vi "TableToXYGraphMot.vi"(1 "Input Table":string[][](array[string])) -> (0 "XY Graph":cluster{"Y":dbl[], "Y":dbl[]}[](graph) caption="Graphe XY")   [LabVIEW 2010]
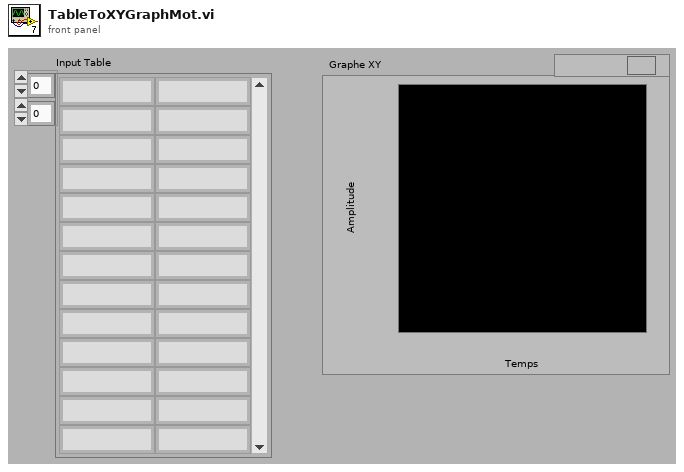
[diagram p1: front panel]
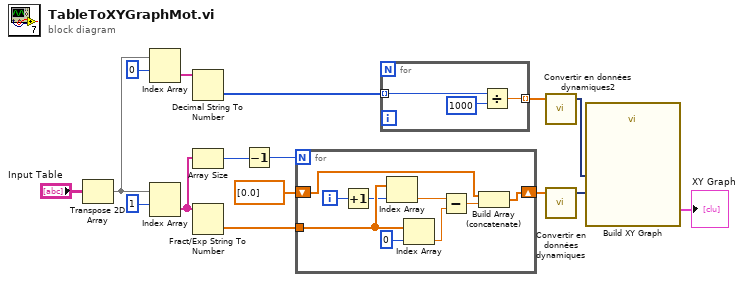
[diagram p0: block diagram]
diagram:
  n1 = Transpose 2D Array(2D array="Input Table") -> (transposed array=w7:string[][])
  n2 = Index Array(array=w7, index (row)=0 ("indice (ligne)")) -> (element=w5:string[])  [unwired: 1 in]
  n3 = Index Array(array=w7, index (row)=1 ("indice (ligne)")) -> (element=w13:string[])  [unwired: 1 in]
  n4 = Decimal String To Number(string=w5) -> (number=w2:i32[])  [unwired: 2 in, 1 out]
  n5 = Array Size(array=w13) -> (size(s)=w14:i32)
  n6 = Fract/Exp String To Number(string=w13) -> (number=w11:dbl[])  [unwired: 3 in, 1 out]
  n7 = Decrement(x=w14) -> (x-1=w15:i32)
  n8 = for {
    N: w15 -> [_]
    tunnel: w11 -> [w25]
    shift-right: [w18] -> w16
    shift-left: dbl[] [0.0] -> [w19]
    i -> [w24]
    n9 = Increment(x=w24) -> (x+1=w23:i32)
    n10 = Index Array(array=w25, index=w23) -> (element=w21:dbl)
    n11 = Index Array(array=w25, index=0 ("indice")) -> (element=w20:dbl)
    n12 = Subtract(x=w21, y=w20) -> (x-y=w17:dbl)
    n13 = Build Array (concatenate)(w19, w17) -> (w18:dbl[])
  }
  n14 = for {
    tunnel: w2 -> [w28] mode=indexing
    tunnel: [w26] -> w1 mode=indexing
    n15 = Divide(x=w28, y=1000) -> (x/y=w26:dbl)
  }
  n16 = call "Convertir en données dynamiques2"("Array"=w1) -> ("Dynamic Data Type"=w3:dynamicdata)  [unwired: 3 in]
  n17 = call "Convertir en données dynamiques"("Array"=w16) -> ("Dynamic Data Type"=w4:dynamicdata)  [unwired: 3 in]
  n18 = call "Build XY Graph"("Y Input"=w4, "X Input"=w3) -> ("XY Graph"=→"XY Graph":cluster{"Y":dbl[], "Y":dbl[]}[])  [unwired: 3 in, 6 out]
